vi "Triggering.vi"() -> ()   [LabVIEW 2011]
uses:
  <vilib>/DAQmx/read.llb/DAQmx Read (Analog Wfm 1Chan NSamp).vi
  <vilib>/DAQmx/create/channels.llb/DAQmx Create Channel (AI-Voltage-Basic).vi
  <vilib>/DAQmx/configure/timing.llb/DAQmx Timing (Sample Clock).vi
  <vilib>/DAQmx/configure/trigger.llb/DAQmx Start Trigger (Digital Edge).vi
  <vilib>/Waveform/WDTFileIO.llb/Export Waveform To Spreadsheet File.vi
  <vilib>/DAQmx/miscellaneous.llb/DAQmx Fill In Error Info.vi
panel:
  out "error out":errorcluster
  out "Waveform Graph":waveform(dbl)(graph)
  in  "timeout":dbl=10.0 format="%0.2f"
  in  "source":tag
  in  "edge":i32(ring)=10280 items=["Rising"=10280, "Falling"=10171]
  in  "samples per channel":i32=1000
  in  "rate":dbl=1000.0 format="%0.2f"
  in  "physical channels":tag
  in  "maximum value":dbl=5.0 format="%0.2f"
  in  "minimum value":dbl=-5.0 format="%0.2f"
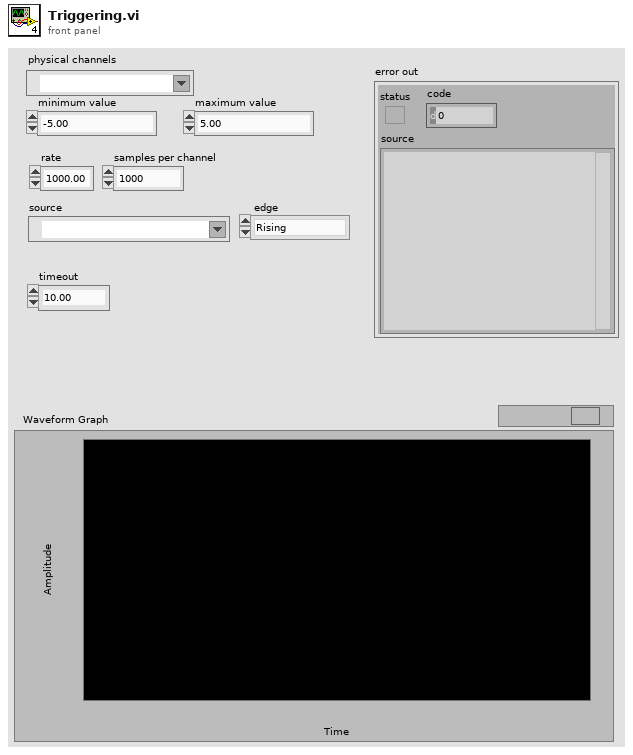
[diagram p1: front panel]
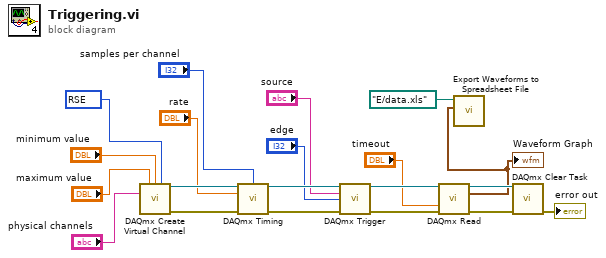
[diagram p0: block diagram]
diagram:
  w18 = 10083 items=["default"=-1, "RSE"=10083, "NRSE"=10078, "Differential"=10106, "Pseudodifferential"=12529] ("input terminal configuration")
  n1 = call-poly <vilib>:"DAQmx Create Virtual Channel.vi"("maximum value"="maximum value", "minimum value"="minimum value", "input terminal configuration"=w18, "physical channels"="physical channels") -> ("task out"=w16:refnum<k21>, "error out"=w15:errorcluster)  [unwired: 10 in]
  n2 = call-poly <vilib>:"DAQmx Timing.vi"("task/channels in"=w16, "samples per channel"="samples per channel", "rate"="rate", "error in"=w15) -> ("task out"=w12:refnum<k21>, "error out"=w11:errorcluster)  [unwired: 10 in]
  n3 = call-poly <vilib>:"DAQmx Trigger.vi"("task/channels in"=w12, "source"="source", "edge"="edge", "error in"=w11) -> ("task out"=w8:refnum<k21>, "error out"=w7:errorcluster)  [unwired: 10 in]
  n4 = call-poly <vilib>:"DAQmx Read.vi"("task/channels in"=w8, "timeout"="timeout", "error in"=w7) -> ("task out"=w5:refnum<k21>, "data"=w2:waveform(dbl), "error out"=w4:errorcluster)  [unwired: 10 in]
  "Waveform Graph" <- w2
  n5 = call-poly <vilib>:"Export Waveforms to Spreadsheet File.vi"("waveform"=w2, "file path (dialog if empty)"=path "E:/data.xls") -> ()  [unwired: 8 in, 2 out]
  n6 = call <vilib>:"DAQmx Clear Task.vi"("task in"=w5, "error in"=w4) -> ("error out"=→"error out":errorcluster)  [unwired: 13 in]
